vi "TestforEXETemplate.vi"() -> ()   [LabVIEW 2016, in "TestLibrary.lvlib"]
uses:
  TestLibrary.lvlib
  <vilib>/SLL Drona/Drona.lvlib
panel:
  out "error out":errorcluster
  in  "EXE Path":path
  in  "Drona Tests PPL":path
  in  "error in (no error)":errorcluster
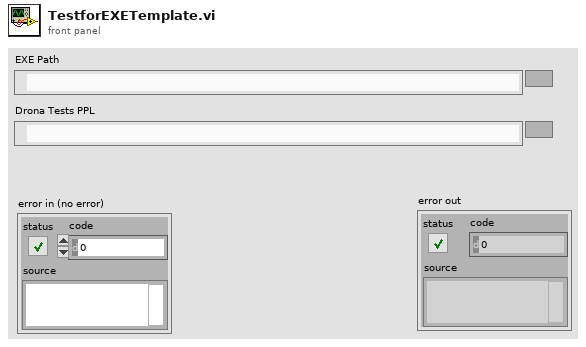
[diagram p1: front panel]
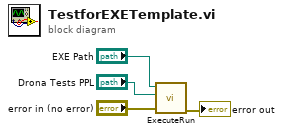
[diagram p0: block diagram]
diagram:
  n1 = call <vilib>:"ExecuteRun.vi"("error in (no error)"="error in (no error)", "Drona Tests PPL"="Drona Tests PPL", "EXE Path"="EXE Path") -> ("error out"=→"error out":errorcluster)  [unwired: 8 in]
